vi "FaceLocationsToRect.vi"(8 "error in (no error)":errorcluster, 11 "FaceLocations":refnum<k24>) -> (0 "error out":errorcluster, 1 "Locations":T1[](array[typedef]), 3 "FaceLocations out":refnum<k24>)   [LabVIEW 2020, in "FaceRecognitionDotNet.lvlib" / "FaceRecognition.lvclass"]
uses:
  FaceRecognition.lvclass
  ctl/Location.ctl
  dll/FaceRecognitionDotNet.dll
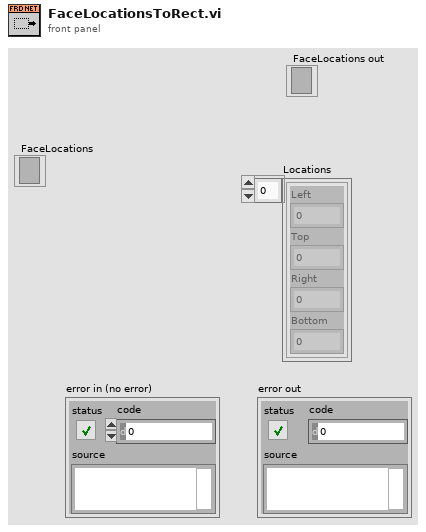
[diagram p1: front panel]
types:
  T1 = typedef "FaceRecognitionDotNet.lvlib/FaceRecognition.lvclass/Location.ctl" = cluster{"Left":i32, "Top":i32, "Right":i32, "Bottom":i32}
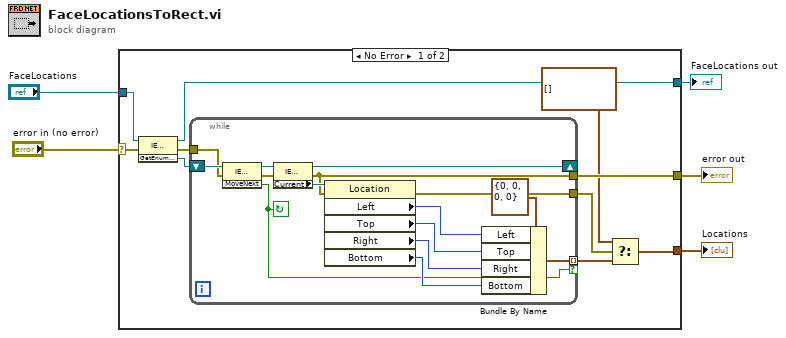
[diagram p0: block diagram]
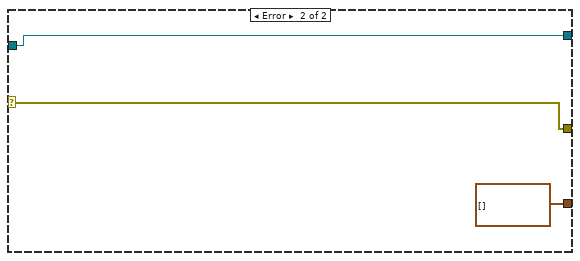
[diagram p2: hidden frame]
diagram:
  n1 = case shown="No Error" "error in (no error)" {
    selector: "error in (no error)" -> [w11 w32]
    tunnel: "FaceLocations" -> [w15 w31]
    tunnel: [w7 T1[] []] -> w4
    tunnel: [w12 w32] -> w3
    tunnel: [w6 w31] -> w1
    frame No Error {
      n2 = invoke class="IEnumerable`1[[FaceRecognitionD" method="GetEnumerator"(reference=w15, error in=w11) -> (reference out=w6:refnum<k24>, error out=w13:errorcluster, "GetEnumerator"=w14:refnum<k24>)  [unwired: 1 in]
      n3 = while {
        shift-right: [w23] -> _
        shift-left: w14 -> [w30]
        tunnel: w13 -> [w22]
        tunnel: [w19] -> w12
        tunnel: [w20] -> w9 mode=indexing if=w16
        tunnel: [w17] -> w10
        stop <- w16 continue-if-true
        n4 = invoke class="IEnumerator`1[[FaceRecognitionD" method="MoveNext"(reference=w30, error in=w22) -> (reference out=w29:refnum<k24>, error out=w21:errorcluster, "MoveNext"=w16:bool)  [unwired: 1 in]
        n5 = property class="IEnumerator`1[[FaceRecognitionD"(reference=w29, error in=w21) -> (reference out=w23:refnum<k24>, error out=w19:errorcluster, "Current"=w28:refnum<k24>)
        n6 = property class="Location"(reference=w28, error in=w19) -> (error out=w17:errorcluster, "Left"=w24:i32, "Top"=w25:i32, "Right"=w26:i32, "Bottom"=w27:i32)  [unwired: 1 out]
        n7 = Bundle By Name(cluster=T1 {"Left"=0, "Top"=0, "Right"=0, "Bottom"=0} ("Rectangle"), "Left"=w24, "Top"=w25, "Right"=w26, "Bottom"=w27) -> (w20:T1)
      }
      n8 = Select(t=T1[] [], s=w10, f=w9) -> (s? t:f=w7:T1[])
    }
    frame Error {
    }
  }
  "Locations" <- w4
  "error out" <- w3
  "FaceLocations out" <- w1
